vi "Telop Bo Peep Begin.vi"   [LabVIEW 2014]
uses:
  <vilib>/Rock Robotics/WPI/Solenoid/WPI_SolenoidValue.ctl
  Robot Global Data.vi
  <vilib>/Rock Robotics/WPI/Solenoid/WPI_SolenoidSetEnum.vi
types:
  T1 = typedef "WPI_SolenoidValue.ctl" = enum16{"Off", "On", "Forward", "Reverse"}
  T2 = typedef "WPI_SolenoidDevRef.ctl" = cluster{"DevStatus":errorcluster, "Pneumatics Control Module":u8, "Forward Solenoid Channel":T3, "Reverse Solenoid Channel":T3}
  T3 = typedef "WPI_SolenoidChannel.ctl" = enum8{"Solenoid 0", "Solenoid 1", "Solenoid 2", "Solenoid 3", "Solenoid 4", "Solenoid 5", "Solenoid 6", "Solenoid 7", "Invalid"}
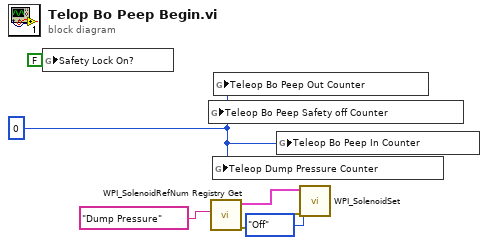
[diagram p0: block diagram]
diagram:
  w5 = i8 0 ("Teleop Bo Peep Out Counter")
  n1 = global write "Robot Global Data.vi" "Safety Lock On?"(FALSE ("Safety Lock On?")) -> ()
  n2 = global write "Robot Global Data.vi" "Teleop Bo Peep Safety off Counter"(w5) -> ()
  n3 = call <vilib>:"WPI_SolenoidRefNum Registry Get.vi"("refnum name"="Dump Pressure") -> ("error out"=w4:errorcluster, "SolenoidDevRef"=w3:T2)  [unwired: 9 in]
  n4 = global write "Robot Global Data.vi" "Teleop Dump Pressure Counter"(w5) -> ()
  n5 = global write "Robot Global Data.vi" "Teleop Bo Peep Out Counter"(w5) -> ()
  n6 = global write "Robot Global Data.vi" "Teleop Bo Peep In Counter"(w5) -> ()
  n7 = call-poly <vilib>:"WPI_SolenoidSet.vi"("error in (no error)"=w4, "Value"=WPI_SolenoidValue."Off", "SolenoidDevRef"=w3) -> ()  [unwired: 7 in, 2 out]
